vi "Riccati_Input_Check.vi"(8 "R":T1, 9 "Q":T1, 10 "B":T1, 11 "A":T1) -> (3 "Error":bool)   [LabVIEW 2019, in "Trajectory_Library.lvlib"]
uses:
  Trajectory_Library.lvlib
  <vilib>/Analysis/Matrix/Datatypes/RealMatrix.ctl
  <vilib>/Analysis/7linalg.llb/Eigenvalue and Vectors Output Option.ctl
  <vilib>/Analysis/7linalg.llb/Real Cholesky Factorization.vi
  <vilib>/Analysis/baseanly.llb/Full Cholesky Factorization.vi
  <vilib>/Analysis/baseanly.llb/Full Real Matrix Cholesky Factorization.vi
  <vilib>/Analysis/7linalg.llb/Real Eigenvalues and Vectors.vi
  <vilib>/Analysis/NI_AALPro.lvlib
  <vilib>/Analysis/Matrix/NI_Matrix.lvlib
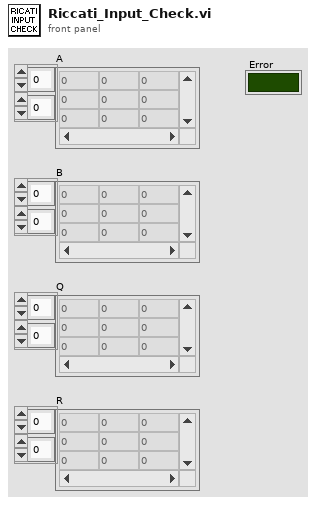
[diagram p1: front panel]
types:
  T1 = typedef "NI_Matrix.lvlib/RealMatrix.ctl" = dbl[][]
  T2 = typedef "NI_AALPro.lvlib/Eigenvalue and Vectors Output Option.ctl" = i32
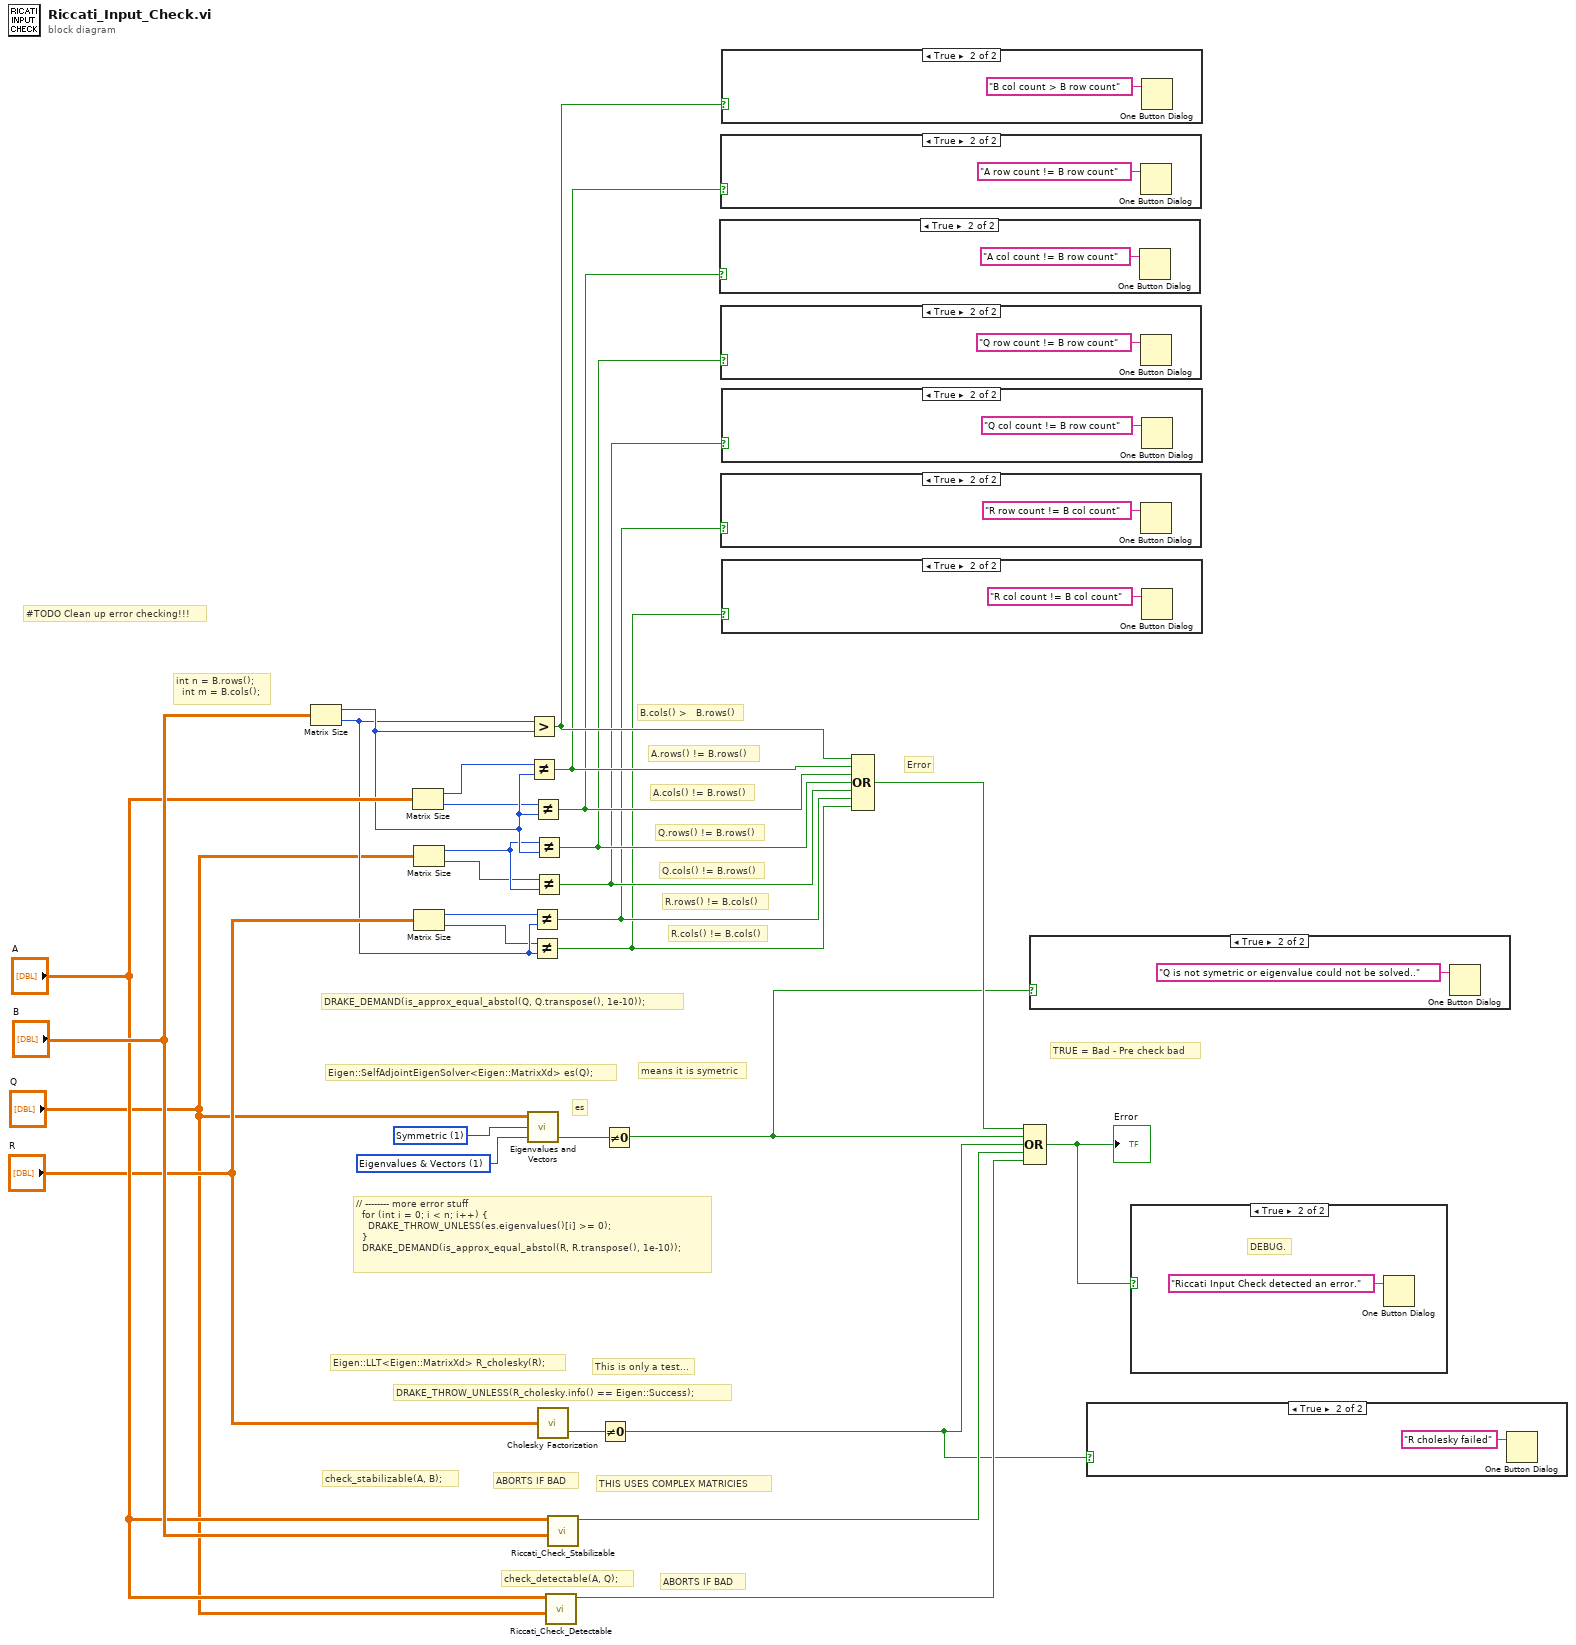
[diagram p0: block diagram]
diagram:
  w14 = 1 items=["General", "Symmetric"] ("matrix type")
  w13 = T2 1 items=["Eigenvalues", "Eigenvalues & Vectors"] ("output option")
  # "R.cols() != B.cols()"
  # "R.rows() != B.cols()"
  # "Q.cols() != B.rows()"
  # "Q.rows() != B.rows()"
  # "A.cols() != B.rows()"
  # "A.rows() != B.rows()"
  # "B.cols() >   B.rows()"
  # "Error"
  # "#TODO Clean up error checking!!!"
  # "TRUE = Bad - Pre check bad"
  # "DRAKE_DEMAND(is_approx_equal_abstol(Q, Q.transpose(), 1e-10));"
  # "int n = B.rows(); \n  int m = B.cols();"
  # "This is only a test..."
  # "ABORTS IF BAD"
  # "ABORTS IF BAD"
  # "check_stabilizable(A, B);"
  # "THIS USES COMPLEX MATRICIES"
  # "DRAKE_THROW_UNLESS(R_cholesky.info() == Eigen::Success);"
  # "// -------- more error stuff\n  for (int i = 0; i < n; i++) {\n    DRAKE_THROW_UNLESS(es.eigenvalues()[i] >= 0);\n  }\n  DRAKE_DEMAND(is_approx_equal_abstol(R, R.transpose(), 1e-10));"
  # "check_detectable(A, Q);"
  # "Eigen::LLT<Eigen::MatrixXd> R_cholesky(R);"
  # "es"
  # "means it is symetric"
  # "Eigen::SelfAdjointEigenSolver<Eigen::MatrixXd> es(Q);"
  n1 = Matrix Size(0:"B") -> (1:w22:i32, 2:w21:i32)
  n2 = Matrix Size(0:"A") -> (1:w15:i32, 2:w16:i32)
  n3 = Matrix Size(0:"Q") -> (1:w18:i32, 2:w17:i32)
  n4 = Matrix Size(0:"R") -> (1:w19:i32, 2:w20:i32)
  n5 = call-poly <vilib>:"Eigenvalues and Vectors.vi"("output option"=w13, "matrix type"=w14, "Input Matrix"="Q") -> ("error"=w24:i32)  [unwired: 2 out]
  n6 = Greater?(x=w21, y=w22) -> (0:w9:bool)
  n7 = Not Equal?(x=w15, y=w22) -> (x != y?=w8:bool)
  n8 = Not Equal?(x=w19, y=w21) -> (x != y?=w4:bool)
  n9 = Not Equal?(x=w20, y=w21) -> (x != y?=w3:bool)
  n10 = Not Equal?(x=w16, y=w22) -> (x != y?=w7:bool)
  n11 = Not Equal?(x=w18, y=w22) -> (x != y?=w6:bool)
  n12 = Not Equal?(x=w17, y=w18) -> (x != y?=w5:bool)
  n13 = call-poly <vilib>:"Cholesky Factorization.vi"("A"="R") -> ("error"=w23:i32)  [unwired: 1 out]
  n14 = call "Riccati_Check_Detectable.vi"("Q"="Q", "A"="A") -> ("Bad"=w26:bool)  [unwired: 9 in]
  n15 = call "Riccati_Check_Stabilizable.vi"("B"="B", "A"="A") -> ("Bad"=w25:bool)  [unwired: 9 in]
  n16 = Not Equal To 0?(x=w23) -> (x != 0?=w1:bool)
  n17 = Not Equal To 0?(x=w24) -> (x != 0?=w2:bool)
  n18 = case shown="True" w7 {
    frame False {
    }
    frame True {
      n19 = One Button Dialog(message="A col count != B row count") -> ()  [unwired: 1 in, 1 out]
    }
  }
  n20 = case shown="True" w8 {
    frame False {
    }
    frame True {
      n21 = One Button Dialog(message="A row count != B row count") -> ()  [unwired: 1 in, 1 out]
    }
  }
  n22 = case shown="True" w6 {
    frame False {
    }
    frame True {
      n23 = One Button Dialog(message="Q row count != B row count") -> ()  [unwired: 1 in, 1 out]
    }
  }
  n24 = case shown="True" w4 {
    frame False {
    }
    frame True {
      n25 = One Button Dialog(message="R row count != B col count") -> ()  [unwired: 1 in, 1 out]
    }
  }
  n26 = case shown="True" w9 {
    frame False {
    }
    frame True {
      n27 = One Button Dialog(message="B col count > B row count") -> ()  [unwired: 1 in, 1 out]
    }
  }
  n28 = case shown="True" w5 {
    frame False {
    }
    frame True {
      n29 = One Button Dialog(message="Q col count != B row count") -> ()  [unwired: 1 in, 1 out]
    }
  }
  n30 = case shown="True" w3 {
    frame False {
    }
    frame True {
      n31 = One Button Dialog(message="R col count != B col count") -> ()  [unwired: 1 in, 1 out]
    }
  }
  n32 = Compound Arithmetic op=OR(w9, w8, w7, w6, w5, w4, w3) -> (w10:bool)
  n33 = Compound Arithmetic op=OR(w10, w2, w1, w25, w26) -> (w11:bool)
  "Error" <- w11
  n34 = case shown="True" w2 {
    frame False {
    }
    frame True {
      n35 = One Button Dialog(message="Q is not symetric or eigenvalue could not be solved..") -> ()  [unwired: 1 in, 1 out]
    }
  }
  n36 = case shown="True" w1 {
    frame False {
    }
    frame True {
      n37 = One Button Dialog(message="R cholesky failed") -> ()  [unwired: 1 in, 1 out]
    }
  }
  n38 = case shown="True" w11 {
    frame False {
    }
    frame True {
      # "DEBUG."
      n39 = One Button Dialog(message="Riccati Input Check detected an error.") -> ()  [unwired: 1 in, 1 out]
    }
  }
